vi "Home.vi"   [LabVIEW 2019]
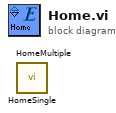
[diagram p0: block diagram]
diagram:
  n1 = call "HomeMultiple.vi"() -> ()  [unwired: 10 in, 2 out]
  n2 = call "HomeSingle.vi"() -> ()  [unwired: 10 in, 2 out]
